vi "Testes 03.02.vi"() -> ()   [LabVIEW 2025]
uses:
  <vilib>/DAQmx/read.llb/DAQmx Read (Counter U32 1Chan 1Samp).vi
  <vilib>/DAQmx/read.llb/DAQmx Read (Analog Wfm 1Chan NSamp).vi
  <vilib>/DAQmx/write.llb/DAQmx Write (Digital Bool 1Line 1Point).vi
  <vilib>/DAQmx/create/channels.llb/DAQmx Create Channel (CO-Pulse Generation-Frequency).vi
  <vilib>/DAQmx/configure/timing.llb/DAQmx Timing (Implicit).vi
  <vilib>/DAQmx/create/channels.llb/DAQmx Create Channel (DO-Digital Output).vi
  <vilib>/DAQmx/miscellaneous.llb/DAQmx Fill In Error Info.vi
  <vilib>/DAQmx/create/channels.llb/DAQmx Create Channel (AI-Voltage-Basic).vi
  <vilib>/DAQmx/configure/timing.llb/DAQmx Timing (Sample Clock).vi
  <vilib>/DAQmx/create/channels.llb/DAQmx Create Channel (CI-Count Edges).vi
  <vilib>/Waveform/WDTFileIO.llb/Export Waveform To Spreadsheet File.vi
  <resource>/objmgr/daqmx.rc
panel:
  in  "Tab Control 2":enum32{"Page 1", "Page 2"}(tab)
  out "Waveform Graph":waveform(dbl)(graph)
  out "Distância (mm)":u32
  out "Numeric":i32
  in  "stop 2":bool
  in  "Path":path
  in  "append to file? (new file:F)":bool=TRUE
  in  "Salvar Dados":bool
  in  "Tab Control":enum32{"Page 1", "Page 2"}(tab)
  in  "Enable":bool
  in  "Distancia (mm)":dbl
  in  "Constante Calibracao (mm/pulsos)":dbl
  in  "Velocidade ( mm/s )":dbl
  in  "stop":bool
  in  "Direção":bool
  out "Elapsed Time (s)":dbl
  out "Loop Count":i32
  in  "Timer Reset":bool
  in  "Pulso":tag
  in  "Direção":tag
  in  "Enable":tag
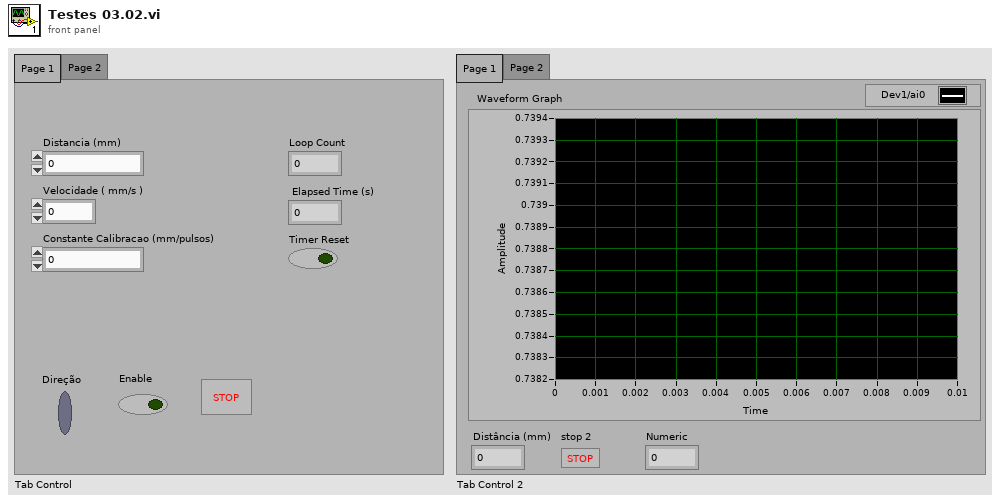
[diagram p1: front panel]
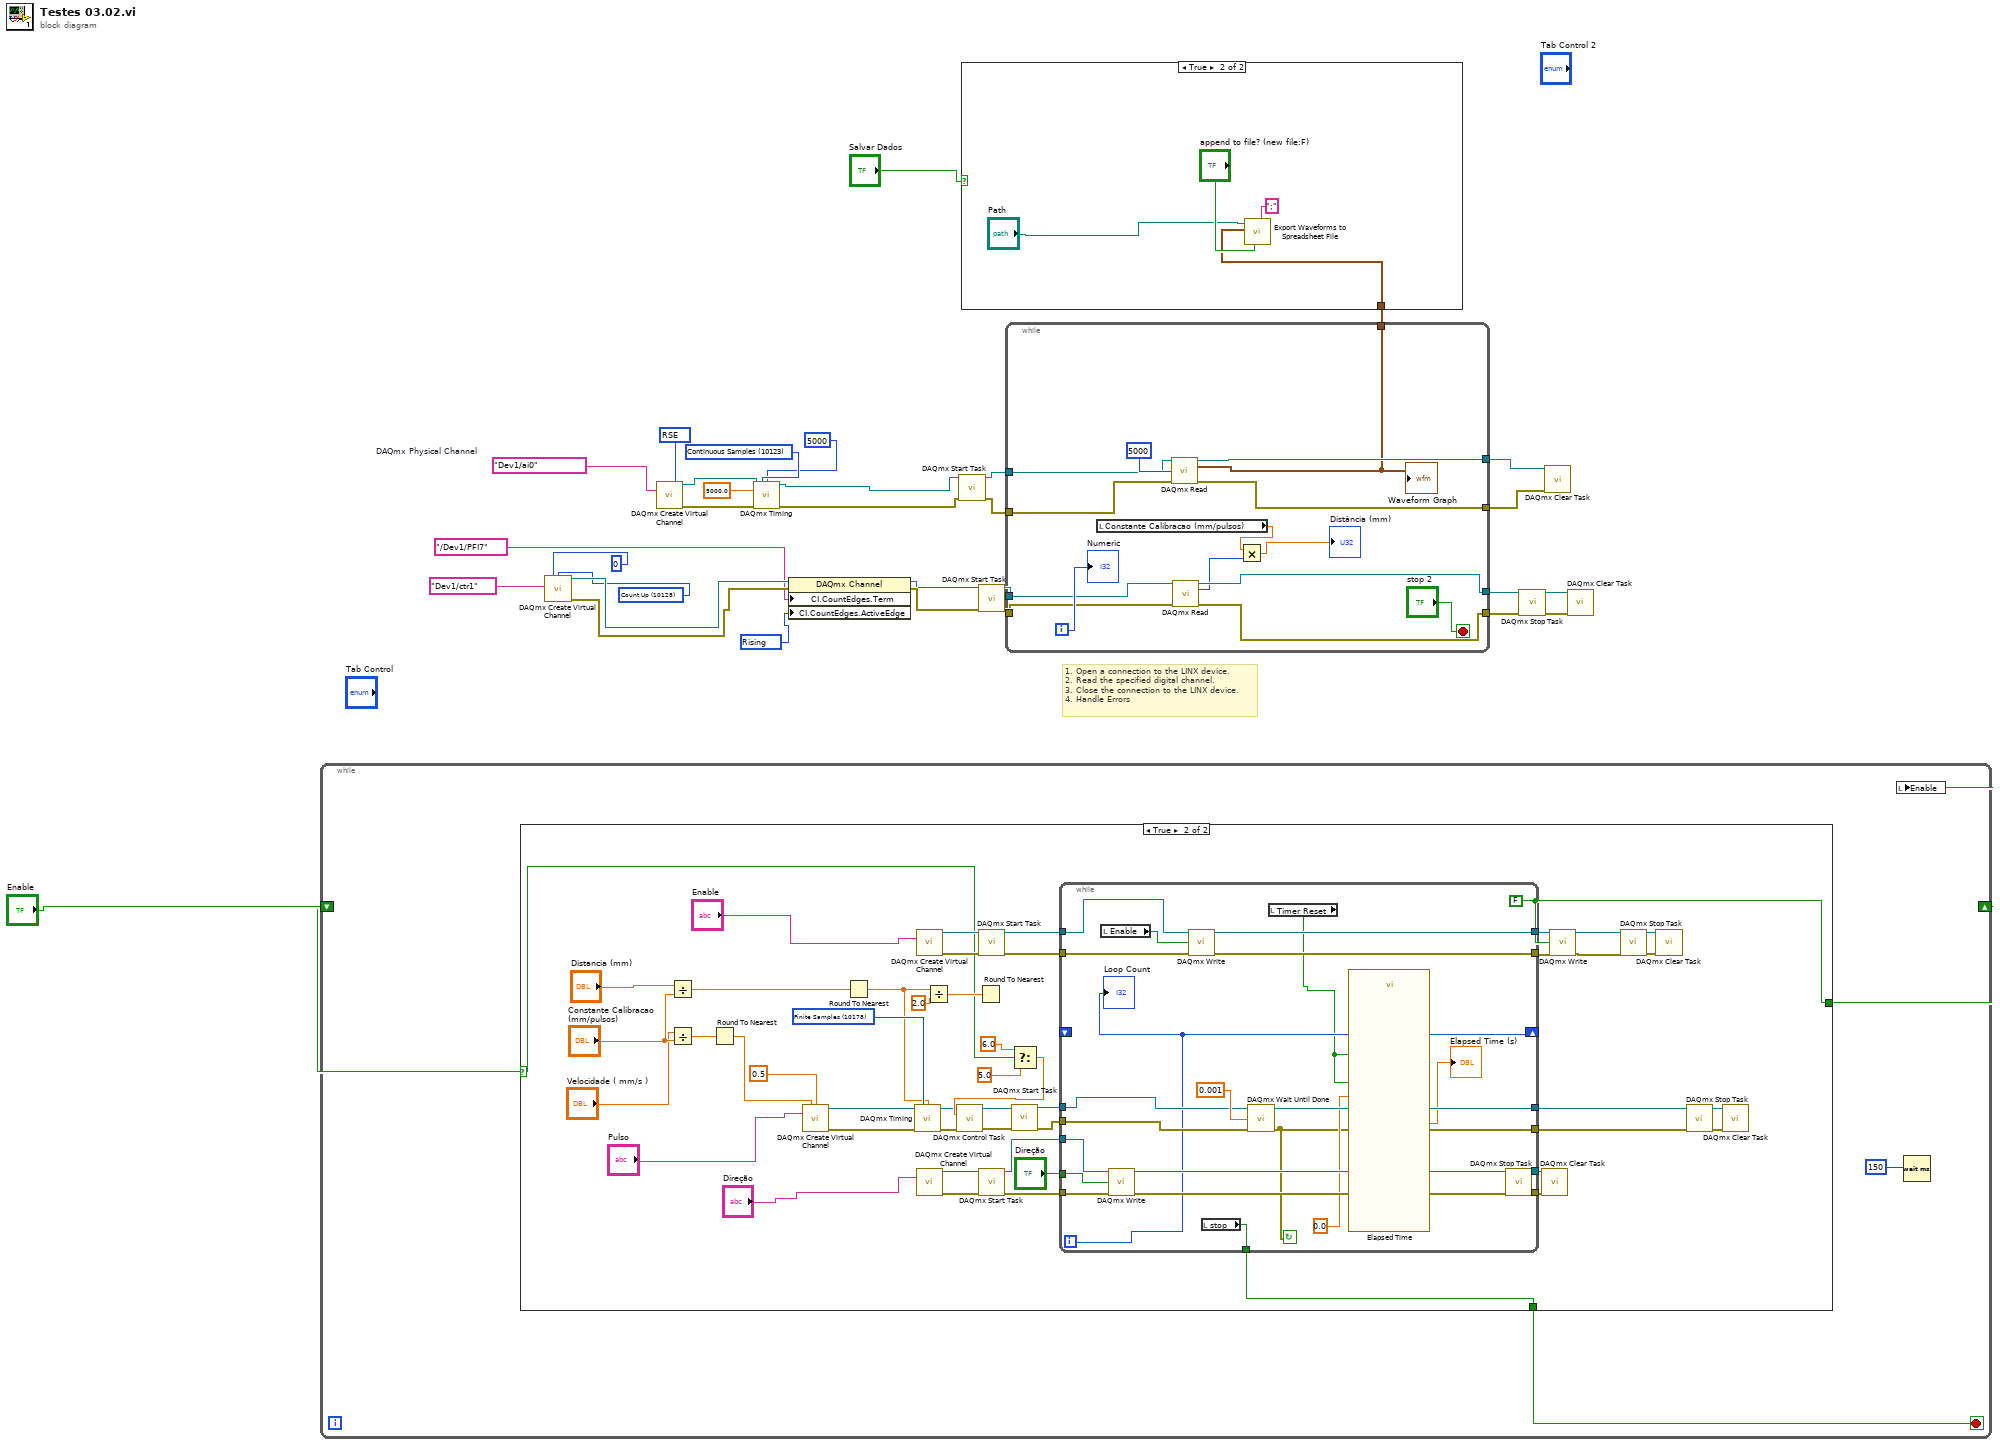
[diagram p0: block diagram]
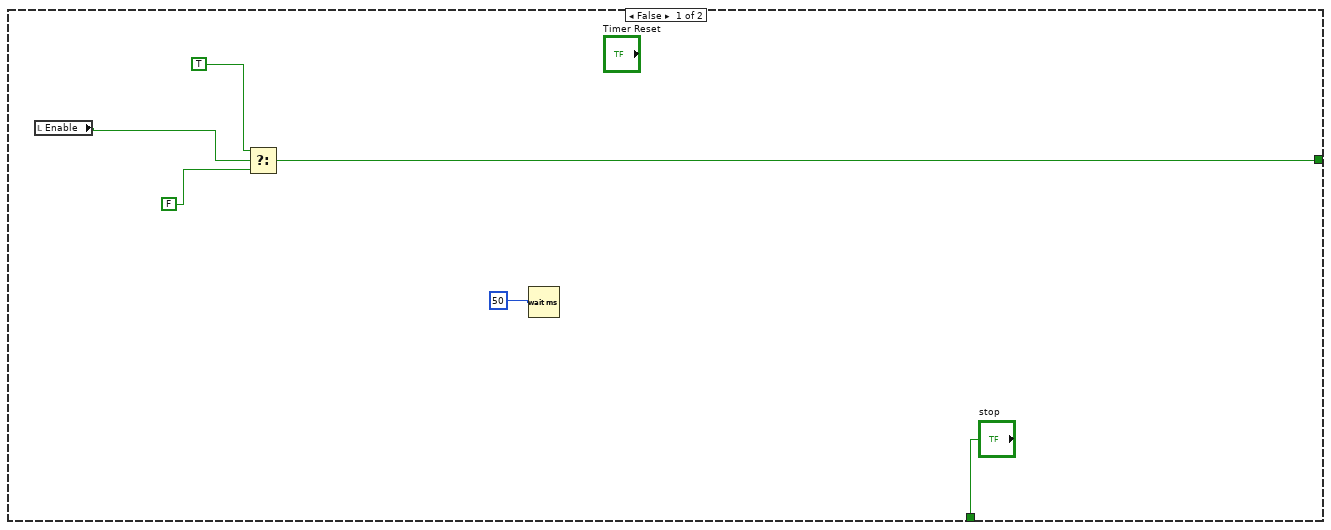
[diagram p3: hidden frame]
diagram:
  w11 = 10280 items=["Rising"=10280, "Falling"=10171] ("CI.CountEdges.ActiveEdge")
  w9 = 10128 items=["Count Up"=10128, "Count Down"=10124, "Externally Controlled"=10326] ("count direction")
  w4 = 10083 items=["Default"=-1, "RSE"=10083, "NRSE"=10078, "Differential"=10106, "Pseudodifferential"=12529] ("input terminal configuration")
  w7 = 10123 items=["Finite Samples"=10178, "Continuous Samples"=10123, "Hardware Timed Single Point"=12522] ("sample mode")
  w3 = tag "Dev1/ai0"  # DAQmx Physical Channel
  # "1. Open a connection to the LINX device.\n2. Read the specified digital channel.\n3. Close the connection to the LINX device.\n4. Handle Errors"
  n1 = while {
    shift-right: [w34] -> _
    shift-left: "Enable" -> [w35]
    stop <- w32 stop-if-true
    n2 = case shown="True" w35 {
      selector: w35 -> [_ w48]
      tunnel: [w37 w43] -> w34
      tunnel: ["stop" w42] -> w32
      frame False {
        n3 = local read "Enable"() -> (w38:bool)
        n4 = Select(t=TRUE, s=w38, f=FALSE) -> (s? t:f=w37:bool)
        n5 = Wait (ms)(milliseconds to wait=u32 50) -> ()  [unwired: 1 out]
      }
      frame True {
        w43 = FALSE ("data")
        w76 = 10178 items=["Finite Samples"=10178, "Continuous Samples"=10123, "Hardware Timed Single Point"=12522] ("sample mode")
        n6 = Divide(x="Distancia (mm)", y="Constante Calibracao (mm/pulsos)") -> (x/y=w68:dbl)
        n7 = Divide(x="Velocidade ( mm/s )", y="Constante Calibracao (mm/pulsos)") -> (x/y=w66:dbl)
        n8 = Round To Nearest(number=w66) -> (nearest integer value=w64:dbl)
        n9 = call-poly <vilib>:"DAQmx Create Virtual Channel.vi"("frequency"=w64, "duty cycle"=0.5, "counter"="Pulso") -> ("task out"=w78:refnum<k21>, "error out"=w77:errorcluster)  [unwired: 11 in]
        n10 = Round To Nearest(number=w68) -> (nearest integer value=w67:dbl)
        n11 = call-poly <vilib>:"DAQmx Timing.vi"("task/channels in"=w78, "sample mode"=w76, "samples per channel"=w67, "error in"=w77) -> ("task out"=w54:refnum<k21>, "error out"=w49:errorcluster)  [unwired: 10 in]
        n12 = call-poly <vilib>:"DAQmx Create Virtual Channel.vi"("lines"="Enable") -> ("task out"=w90:refnum<k21>, "error out"=w91:errorcluster)  [unwired: 13 in]
        n13 = call-poly <vilib>:"DAQmx Create Virtual Channel.vi"("lines"="Direção") -> ("task out"=w92:refnum<k21>, "error out"=w89:errorcluster)  [unwired: 13 in]
        n14 = Divide(x=w67, y=2.0) -> (x/y=w65:dbl)
        n15 = Round To Nearest(number=w65) -> ()  [unwired: 1 out]
        n16 = call <vilib>:"DAQmx Start Task.vi"("task/channels in"=w90, "error in"=w91) -> ("task out"=w86:refnum<k21>, "error out"=w85:errorcluster)  [unwired: 12 in]
        n17 = call <vilib>:"DAQmx Start Task.vi"("task/channels in"=w92, "error in"=w89) -> ("task out"=w88:refnum<k21>, "error out"=w87:errorcluster)  [unwired: 12 in]
        n18 = Select(t=6.0 ("y"), s=w48, f=5.0 ("y")) -> (s? t:f=w55:dbl)
        n19 = call <vilib>:"DAQmx Control Task.vi"("task/channels in"=w54, "action"=w55, "error in"=w49) -> ("task out"=w53:refnum<k21>, "error out"=w50:errorcluster)  [unwired: 11 in]
        n20 = call <vilib>:"DAQmx Start Task.vi"("task/channels in"=w53, "error in"=w50) -> ("task out"=w52:refnum<k21>, "error out"=w51:errorcluster)  [unwired: 12 in]
        n21 = while {
          tunnel: w88 -> [w112]
          tunnel: w87 -> [w111]
          tunnel: w86 -> [w110]
          tunnel: w85 -> [w109]
          tunnel: [w108] -> w80
          tunnel: [w107] -> w79
          tunnel: [w106] -> w46
          tunnel: [w105] -> w44
          tunnel: "Direção" -> [w104]
          tunnel: [w100] -> w62
          tunnel: [w97] -> w61
          shift-right: [w96] -> _
          shift-left: _ -> [_]
          tunnel: w51 -> [w102]
          tunnel: w52 -> [w101]
          tunnel: [w95] -> w42
          i -> [w96]
          stop <- w97 continue-if-true
          n22 = local read "Enable"() -> (w93:bool)
          n23 = call-poly <vilib>:"DAQmx Write.vi"("task/channels in"=w112, "data"=w104, "error in"=w111) -> ("task out"=w108:refnum<k21>, "error out"=w107:errorcluster)  [unwired: 10 in, 1 out]
          n24 = call-poly <vilib>:"DAQmx Write.vi"("task/channels in"=w110, "data"=w93, "error in"=w109) -> ("task out"=w106:refnum<k21>, "error out"=w105:errorcluster)  [unwired: 10 in, 1 out]
          n25 = local read "stop"() -> (w95:bool)
          n26 = call <vilib>:"DAQmx Wait Until Done.vi"("task/channels in"=w101, "timeout (sec)"=0.001 ("y"), "error in"=w102) -> ("task out"=w100:refnum<k21>, "error out"=w97:errorcluster)  [unwired: 11 in]
          n27 = local read "Timer Reset"() -> (w94:bool)
          n28 = call "Elapsed Time"("Reset"=w94, "Auto Reset"=w94, "Set Start Time (s)"=0.0) -> ("Elapsed Time (s)"=→"Elapsed Time (s)":dbl)  [unwired: 9 in, 7 out]
          "Loop Count" <- w96
        }
        n29 = call <vilib>:"DAQmx Stop Task.vi"("task/channels in"=w80, "error in"=w79) -> ("task out"=w84:refnum<k21>, "error out"=w83:errorcluster)  [unwired: 12 in]
        n30 = call <vilib>:"DAQmx Clear Task.vi"("task in"=w84, "error in"=w83) -> ()  [unwired: 13 in, 1 out]
        n31 = call-poly <vilib>:"DAQmx Write.vi"("task/channels in"=w46, "data"=w43, "error in"=w44) -> ("task out"=w47:refnum<k21>, "error out"=w45:errorcluster)  [unwired: 10 in, 1 out]
        n32 = call <vilib>:"DAQmx Stop Task.vi"("task/channels in"=w47, "error in"=w45) -> ("task out"=w82:refnum<k21>, "error out"=w81:errorcluster)  [unwired: 12 in]
        n33 = call <vilib>:"DAQmx Clear Task.vi"("task in"=w82, "error in"=w81) -> ()  [unwired: 13 in, 1 out]
        n34 = call <vilib>:"DAQmx Stop Task.vi"("task/channels in"=w62, "error in"=w61) -> ("task out"=w74:refnum<k21>, "error out"=w73:errorcluster)  [unwired: 12 in]
        n35 = call <vilib>:"DAQmx Clear Task.vi"("task in"=w74, "error in"=w73) -> ()  [unwired: 13 in, 1 out]
      }
    }
    n36 = local write "Enable"(w34) -> ()
    n37 = Wait (ms)(milliseconds to wait=u32 150) -> ()  [unwired: 1 out]
  }
  n38 = call-poly <vilib>:"DAQmx Create Virtual Channel.vi"("initial count"=u32 0, "count direction"=w9, "counter"=tag "Dev1/ctr1") -> ("task out"=w21:refnum<k21>, "error out"=w22:errorcluster)  [unwired: 11 in]
  n39 = call-poly <vilib>:"DAQmx Create Virtual Channel.vi"("input terminal configuration"=w4, "physical channels"=w3) -> ("task out"=w14:refnum<k21>, "error out"=w15:errorcluster)  [unwired: 12 in]
  n40 = call-poly <vilib>:"DAQmx Timing.vi"("task/channels in"=w14, "sample mode"=w7, "samples per channel"=5000, "rate"=5000.0, "error in"=w15) -> ("task out"=w19:refnum<k21>, "error out"=w20:errorcluster)  [unwired: 9 in]
  n41 = property class="DAQmx Channel"(reference=w21, error in=w22, "CI.CountEdges.Term"=tag "/Dev1/PFI7", "CI.CountEdges.ActiveEdge"=w11) -> (reference out=w23:refnum<k21>, error out=w24:errorcluster)
  n42 = call <vilib>:"DAQmx Start Task.vi"("task/channels in"=w19, "error in"=w20) -> ("task out"=w17:refnum<k21>, "error out"=w18:errorcluster)  [unwired: 12 in]
  n43 = call <vilib>:"DAQmx Start Task.vi"("task/channels in"=w23, "error in"=w24) -> ("task out"=w25:refnum<k21>, "error out"=w26:errorcluster)  [unwired: 12 in]
  n44 = while {
    tunnel: [w126] -> w16
    tunnel: [w127] -> w13
    tunnel: w17 -> [w122]
    tunnel: w18 -> [w121]
    tunnel: w25 -> [w120]
    tunnel: w26 -> [w119]
    tunnel: [w118] -> w29
    tunnel: [w117] -> w30
    tunnel: [w113] -> w2
    i -> [w123]
    stop <- "stop 2" stop-if-true
    n45 = local read "Constante Calibracao (mm/pulsos)"() -> (w114:dbl)
    n46 = call-poly <vilib>:"DAQmx Read.vi"("task/channels in"=w122, "number of samples per channel"=5000, "error in"=w121) -> ("task out"=w127:refnum<k21>, "data"=w113:waveform(dbl), "error out"=w126:errorcluster)  [unwired: 10 in]
    "Waveform Graph" <- w113
    n47 = call-poly <vilib>:"DAQmx Read.vi"("task/channels in"=w120, "error in"=w119) -> ("task out"=w118:refnum<k21>, "data"=w116:u32, "error out"=w117:errorcluster)  [unwired: 11 in]
    n48 = Multiply(x=w114, y=w116) -> (x*y=→"Distância (mm)":dbl)
    "Numeric" <- w123
  }
  n49 = case shown="True" "Salvar Dados" {
    tunnel: w2 -> [_ w128]
    frame False {
    }
    frame True {
      n50 = call-poly <vilib>:"Export Waveforms to Spreadsheet File.vi"("delimiter (Tab)"=";", "append to file? (new file:F)"="append to file? (new file:F)", "waveform"=w128, "file path (dialog if empty)"="Path") -> ()  [unwired: 6 in, 2 out]
    }
  }
  n51 = call <vilib>:"DAQmx Stop Task.vi"("task/channels in"=w29, "error in"=w30) -> ("task out"=w27:refnum<k21>, "error out"=w28:errorcluster)  [unwired: 12 in]
  n52 = call <vilib>:"DAQmx Clear Task.vi"("task in"=w13, "error in"=w16) -> ()  [unwired: 13 in, 1 out]
  n53 = call <vilib>:"DAQmx Clear Task.vi"("task in"=w27, "error in"=w28) -> ()  [unwired: 13 in, 1 out]
